vi "H3C psw cable 10G QSFP+读写操作.vi"(6 "input_psw":u8[](array[numeric]) format="%.0x", 8 "input_data":u8[](array[numeric]) format="%.0x", 9 "input_mode":string(combo), 10 "Channel":u8 max=5 step=1, 11 "VISA":refnum<visa-resource-name>="COM6") -> (0 "123equal0?":bool, 1 "result":bool, 2 "message":string, 3 "data read":u8[](array[numeric]) format="%.0x")   [LabVIEW 2011]
panel:
  out "page3 128 Bytes":u8[](array[numeric]) format="%.0x"
  out "page2 128 Bytes":u8[](array[numeric]) format="%.0x"
  out "page1 128 Bytes":u8[](array[numeric]) format="%.0x"
  in  "address":u8
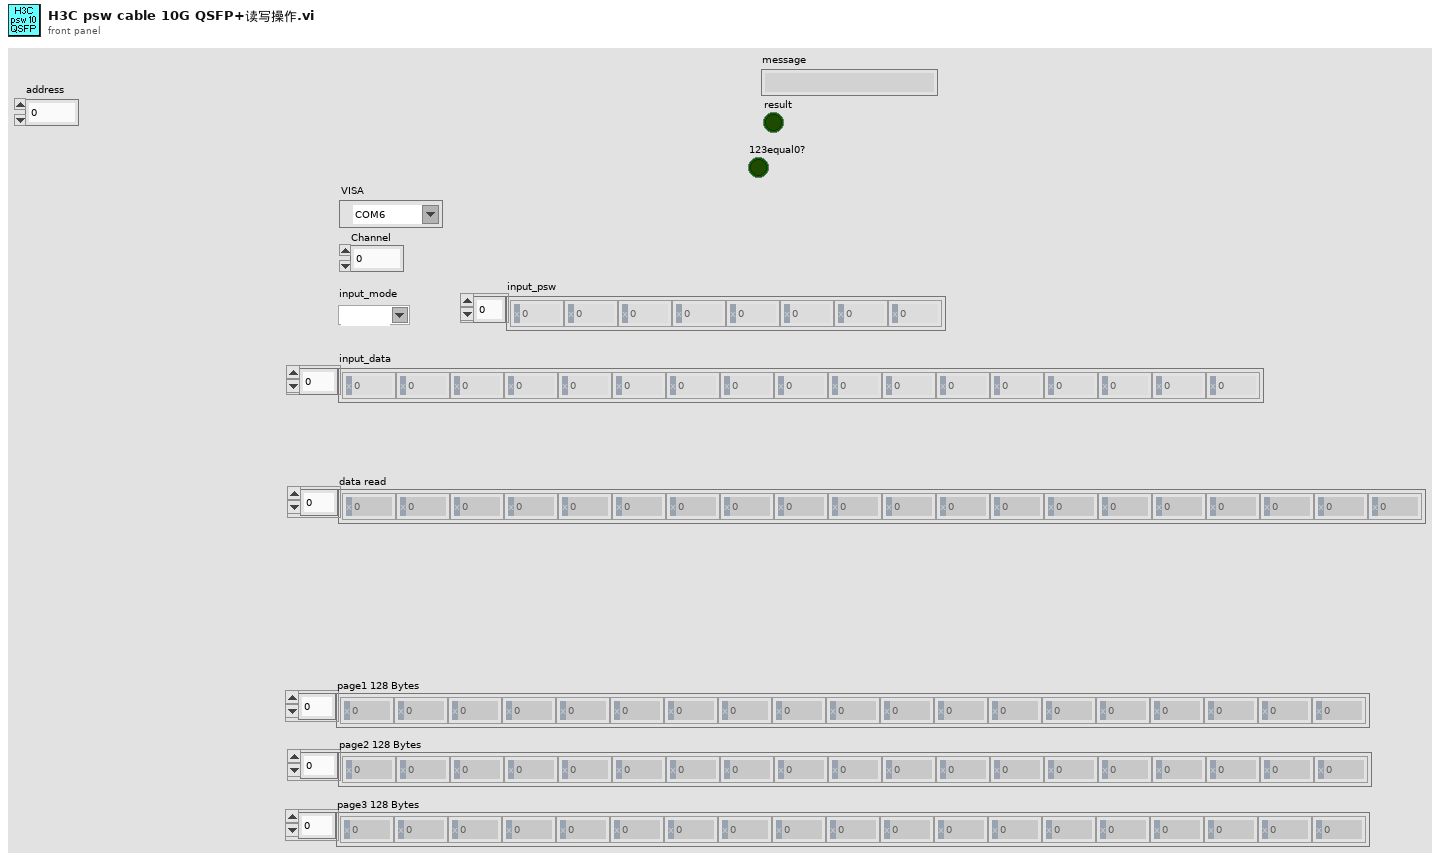
[diagram p1: front panel]
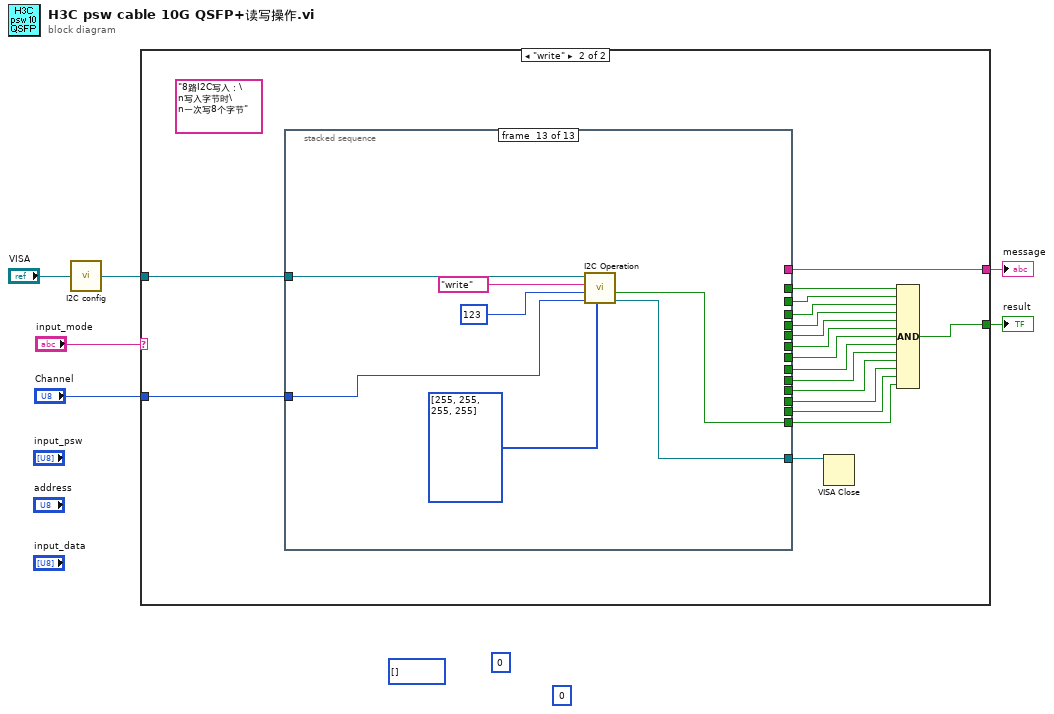
[diagram p0: block diagram]
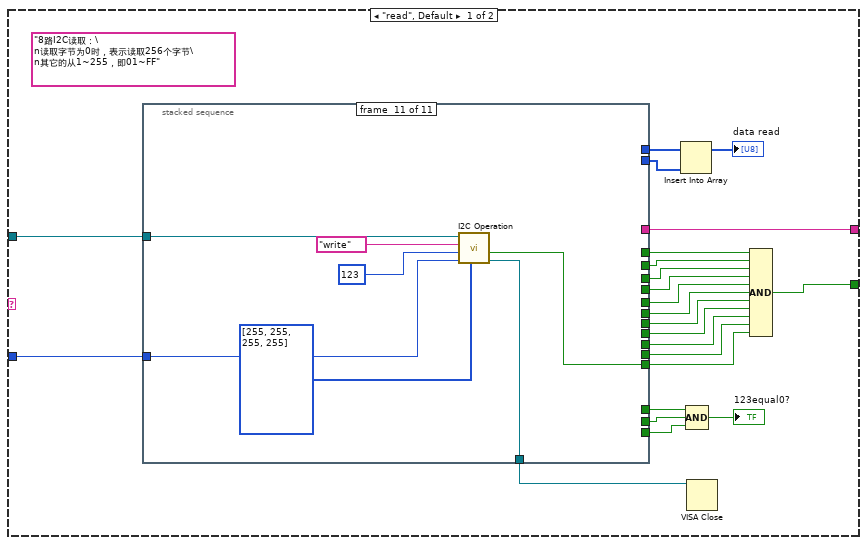
[diagram p2: hidden frame]
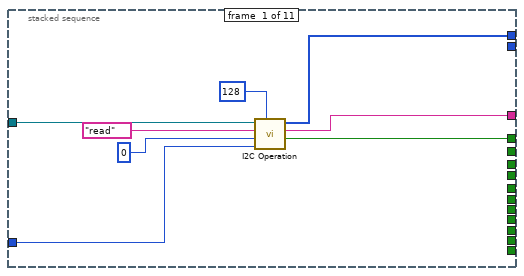
[diagram p3: hidden frame]
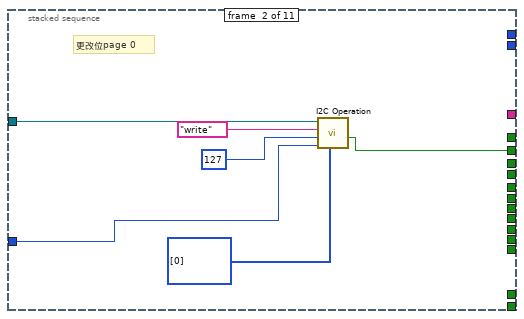
[diagram p4: hidden frame]
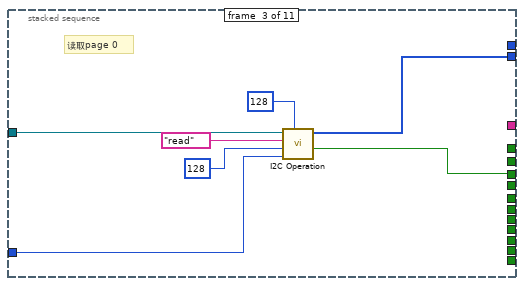
[diagram p5: hidden frame]
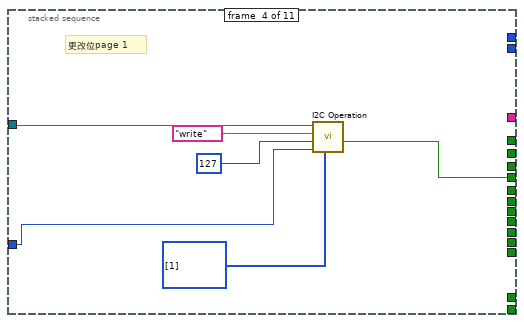
[diagram p6: hidden frame]
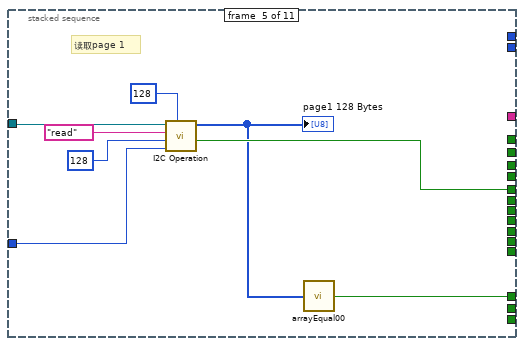
[diagram p7: hidden frame]
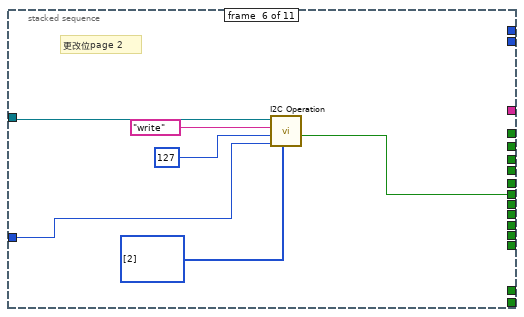
[diagram p8: hidden frame]
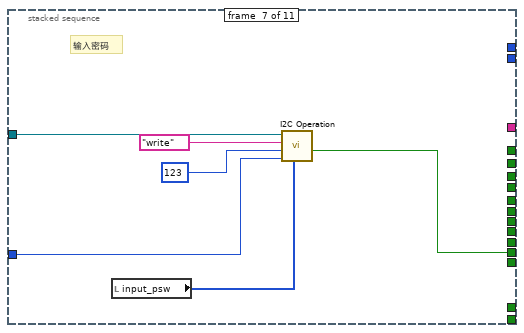
[diagram p9: hidden frame]
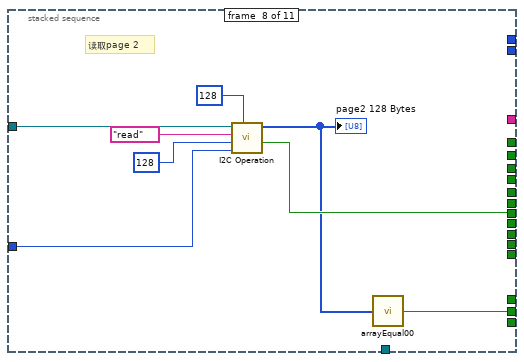
[diagram p10: hidden frame]
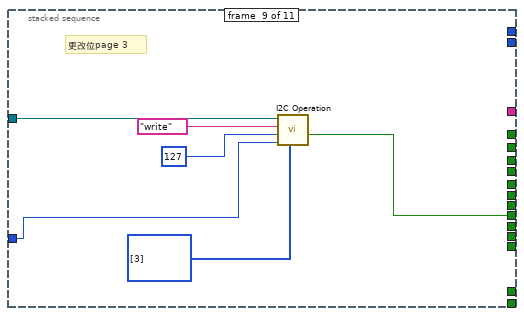
[diagram p11: hidden frame]
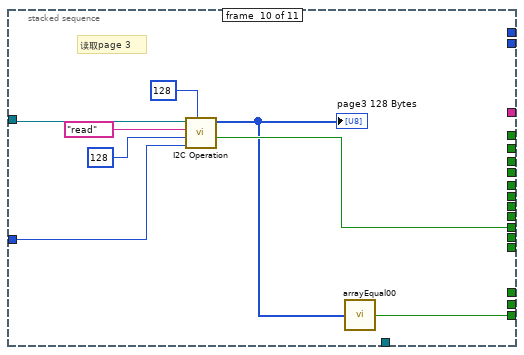
[diagram p12: hidden frame]
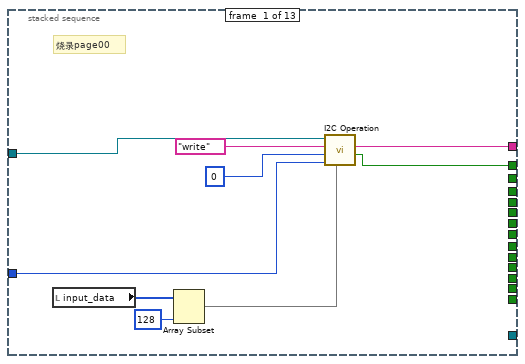
[diagram p13: hidden frame]
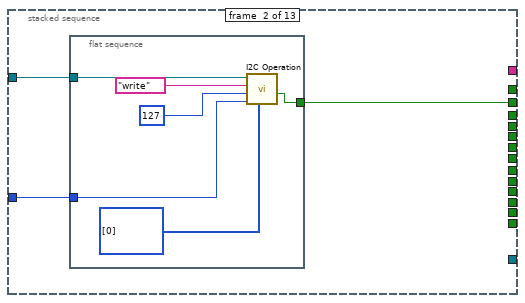
[diagram p14: hidden frame]
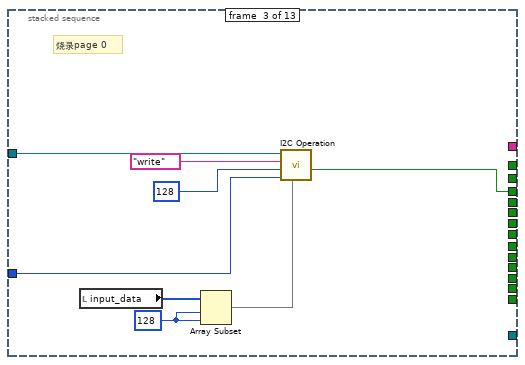
[diagram p15: hidden frame]
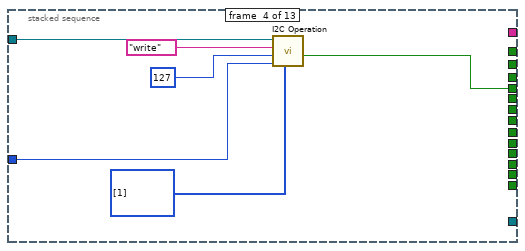
[diagram p16: hidden frame]
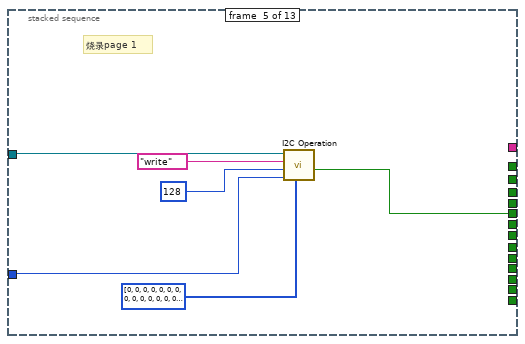
[diagram p17: hidden frame]
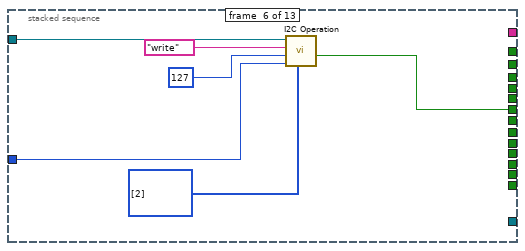
[diagram p18: hidden frame]
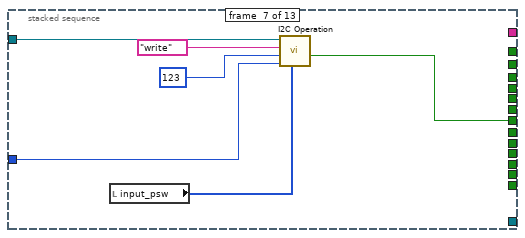
[diagram p19: hidden frame]
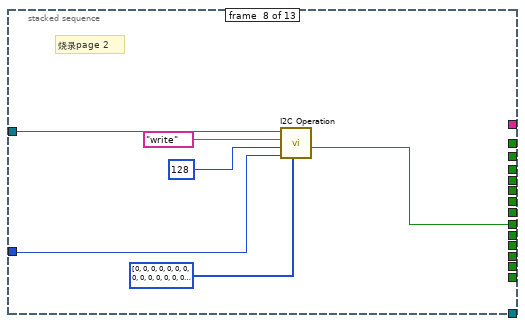
[diagram p20: hidden frame]
diagram:
  (unwired) u8[] []
  (unwired) u8 0
  (unwired) u8 0
  n1 = call "I2C config.vi"("VISA"="VISA") -> ("VISA资源名称输出"=w1:refnum<visa-resource-name>)
  n2 = case shown="\"write\"" "input_mode" {
    tunnel: w1 -> [w29 w123]
    tunnel: "Channel" -> [w28 w122]
    tunnel: [w27 w121] -> w4
    tunnel: [w14 w107] -> w3
    frame "read", Default {
      (unwired) "8路I2C读取：\n读取字节为0时，表示读取256个字节\n其它的从1~255，即01~FF"
      n3 = stacked-sequence {
        tunnel: w29 -> [w37 w40 w50 w53 w61 w67 w73 w81 w87 w95 w103]
        tunnel: w28 -> [w33 w39 w46 w52 w60 w66 w72 w80 w86 w94 w102]
        tunnel: [w32 _ _ _ _ _ _ _ _ _ _] -> w27
        tunnel: [w31 _ _ _ _ _ _ _ _ _ _] -> w23
        tunnel: [w30 _ _ _ _ _ _ _ _ _ _] -> w26
        tunnel: [_ _ w45 _ _ _ _ _ _ _ _] -> w25
        tunnel: [_ w38 _ _ _ _ _ _ _ _ _] -> w22
        tunnel: [_ _ w44 _ _ _ _ _ _ _ _] -> w21
        tunnel: [_ _ _ w51 _ _ _ _ _ _ _] -> w20
        tunnel: [_ _ _ _ w59 _ _ _ _ _ _] -> w19
        tunnel: [_ _ _ _ _ w65 _ _ _ _ _] -> w18
        tunnel: [_ _ _ _ _ _ _ w79 _ _ _] -> w17
        tunnel: [_ _ _ _ _ _ _ _ w85 _ _] -> w16
        tunnel: [_ _ _ _ _ _ _ _ _ w93 _] -> w15
        tunnel: [_ _ _ _ _ _ w71 _ _ _ _] -> w13
        tunnel: [_ _ _ _ _ _ _ _ _ _ w100] -> w12
        tunnel: [_ _ _ _ w57 _ _ _ _ _ _] -> w11
        tunnel: [_ _ _ _ _ _ _ w78 _ _ _] -> w10
        tunnel: [_ _ _ _ _ _ _ _ _ w92 _] -> w9
        tunnel: [_ _ _ _ _ _ _ _ _ _ w99] -> w7
        frame #0 {
          n4 = call "I2C Operation.vi"("size"=128, "Channel"=w33, "address"=u8 0, "mode"="read", "VISA"=w37) -> ("result"=w31:bool, "message"=w32:string, "Data Out"=w30:u8[])  [unwired: 3 in, 1 out]
        }
        frame #1 {
          # "更改位page 0"
          n5 = call "I2C Operation.vi"("input_data"=u8[] [0], "Channel"=w39, "address"=u8 127, "mode"="write", "VISA"=w40) -> ("result"=w38:bool)  [unwired: 3 in, 3 out]
        }
        frame #2 {
          # "读取page 0"
          n6 = call "I2C Operation.vi"("size"=128, "Channel"=w46, "address"=u8 128, "mode"="read", "VISA"=w50) -> ("result"=w44:bool, "Data Out"=w45:u8[])  [unwired: 3 in, 2 out]
        }
        frame #3 {
          # "更改位page 1"
          n7 = call "I2C Operation.vi"("input_data"=u8[] [1], "Channel"=w52, "address"=u8 127, "mode"="write", "VISA"=w53) -> ("result"=w51:bool)  [unwired: 3 in, 3 out]
        }
        frame #4 {
          # "读取page 1"
          n8 = call "I2C Operation.vi"("size"=128, "Channel"=w60, "address"=u8 128, "mode"="read", "VISA"=w61) -> ("result"=w59:bool, "Data Out"=w58:u8[])  [unwired: 3 in, 2 out]
          "page1 128 Bytes" <- w58
          n9 = call "arrayEqual00.vi"("input"=w58) -> ("equal"=w57:bool)
        }
        frame #5 {
          # "更改位page 2"
          n10 = call "I2C Operation.vi"("input_data"=u8[] [2], "Channel"=w66, "address"=u8 127, "mode"="write", "VISA"=w67) -> ("result"=w65:bool)  [unwired: 3 in, 3 out]
        }
        frame #6 {
          # "输入密码"
          n11 = local read "input_psw"() -> (w74:u8[])
          n12 = call "I2C Operation.vi"("input_data"=w74, "Channel"=w72, "address"=u8 123, "mode"="write", "VISA"=w73) -> ("result"=w71:bool)  [unwired: 3 in, 3 out]
        }
        frame #7 {
          # "读取page 2"
          n13 = call "I2C Operation.vi"("size"=128, "Channel"=w80, "address"=u8 128, "mode"="read", "VISA"=w81) -> ("result"=w79:bool, "Data Out"=w77:u8[])  [unwired: 3 in, 2 out]
          "page2 128 Bytes" <- w77
          n14 = call "arrayEqual00.vi"("input"=w77) -> ("equal"=w78:bool)
        }
        frame #8 {
          # "更改位page 3"
          n15 = call "I2C Operation.vi"("input_data"=u8[] [3], "Channel"=w86, "address"=u8 127, "mode"="write", "VISA"=w87) -> ("result"=w85:bool)  [unwired: 3 in, 3 out]
        }
        frame #9 {
          # "读取page 3"
          n16 = call "I2C Operation.vi"("size"=128, "Channel"=w94, "address"=u8 128, "mode"="read", "VISA"=w95) -> ("result"=w93:bool, "Data Out"=w91:u8[])  [unwired: 3 in, 2 out]
          "page3 128 Bytes" <- w91
          n17 = call "arrayEqual00.vi"("input"=w91) -> ("equal"=w92:bool)
        }
        frame #10 {
          n18 = call "I2C Operation.vi"("input_data"=u8[] [255, 255, 255, 255], "Channel"=w102, "address"=u8 123, "mode"="write", "VISA"=w103) -> ("VISA  2"=w99:refnum<visa-resource-name>, "result"=w100:bool)  [unwired: 3 in, 2 out]
        }
      }
      n19 = Insert Into Array(array=w26, new element=w25) -> (→"data read":u8[])  [unwired: 1 in]
      n20 = Compound Arithmetic op=AND(w11, w10, w9) -> (→"123equal0?":bool)
      n21 = VISA Close(VISA resource name=w7) -> ()  [unwired: 1 in, 1 out]
      n22 = Compound Arithmetic op=AND(w23, w22, w21, w20, w19, w18, w17, w16, w15, w13, w12) -> (w14:bool)
    }
    frame "write" {
      (unwired) "8路I2C写入：\n写入字节时\n一次写8个字节"
      n23 = stacked-sequence {
        tunnel: w123 -> [w132 w135 w149 w151 w158 w164 w170 w176 w181 w188 w195 w201 w208]
        tunnel: w122 -> [w130 w134 w147 w152 w157 w165 w171 w175 w182 w187 w194 w200 w207]
        tunnel: [w129 _ _ _ _ _ _ _ _ _ _ _ _] -> w121
        tunnel: [w128 _ _ _ _ _ _ _ _ _ _ _ _] -> w120
        tunnel: [_ w133 _ _ _ _ _ _ _ _ _ _ _] -> w119
        tunnel: [_ _ w145 _ _ _ _ _ _ _ _ _ _] -> w118
        tunnel: [_ _ _ w150 _ _ _ _ _ _ _ _ _] -> w117
        tunnel: [_ _ _ _ w156 _ _ _ _ _ _ _ _] -> w116
        tunnel: [_ _ _ _ _ w162 _ _ _ _ _ _ _] -> w115
        tunnel: [_ _ _ _ _ _ w168 _ _ _ _ _ _] -> w114
        tunnel: [_ _ _ _ _ _ _ w174 _ _ _ _ _] -> w113
        tunnel: [_ _ _ _ _ _ _ _ w180 _ _ _ _] -> w112
        tunnel: [_ _ _ _ _ _ _ _ _ w186 _ _ _] -> w111
        tunnel: [_ _ _ _ _ _ _ _ _ _ w192 _ _] -> w110
        tunnel: [_ _ _ _ _ _ _ _ _ _ _ w198 _] -> w109
        tunnel: [_ _ _ _ _ _ _ _ _ _ _ _ w205] -> w108
        tunnel: [_ _ _ _ _ _ _ _ _ _ _ _ w204] -> w106
        frame #0 {
          # "烧录page00"
          n24 = local read "input_data"() -> (w126:u8[])
          n25 = Array Subset(array=w126, length=128 ("长度")) -> (w124:u8[])  [unwired: 1 in]
          n26 = call "I2C Operation.vi"("input_data"=w124, "Channel"=w130, "address"=u8 0, "mode"="write", "VISA"=w132) -> ("result"=w128:bool, "message"=w129:string)  [unwired: 3 in, 2 out]
        }
        frame #1 {
          n27 = flat-sequence {
            tunnel: [w136] -> w133
            tunnel: w135 -> [w141]
            tunnel: w134 -> [w139]
            frame #0 {
              n28 = call "I2C Operation.vi"("input_data"=u8[] [0], "Channel"=w139, "address"=u8 127, "mode"="write", "VISA"=w141) -> ("result"=w136:bool)  [unwired: 3 in, 3 out]
            }
          }
        }
        frame #2 {
          w144 = 128 ("长度")
          # "烧录page 0"
          n29 = local read "input_data"() -> (w143:u8[])
          n30 = Array Subset(array=w143, index=w144, length=w144) -> (w142:u8[])
          n31 = call "I2C Operation.vi"("input_data"=w142, "Channel"=w147, "address"=u8 128, "mode"="write", "VISA"=w149) -> ("result"=w145:bool)  [unwired: 3 in, 3 out]
        }
        frame #3 {
          n32 = call "I2C Operation.vi"("input_data"=u8[] [1], "Channel"=w152, "address"=u8 127, "mode"="write", "VISA"=w151) -> ("result"=w150:bool)  [unwired: 3 in, 3 out]
        }
        frame #4 {
          # "烧录page 1"
          n33 = call "I2C Operation.vi"("input_data"=u8[] [0, 0, 0, 0, 0, 0, 0, 0, 0, 0, 0, 0, 0, 0, 0, 0, 0, 0, 0, 0, 0, 0, 0, 0, 0, 0, 0, 0, 0, 0, 0, 0, 0, 0, 0, 0, 0, 0, 0, 0, 0, 0, 0, 0, 0, 0, 0, 0, 0, 0, 0, 0, 0, 0, 0, 0, 0, 0, 0, 0, 0, 0, 0, 0, 0, 0, 0, 0, 0, 0, 0, 0, 0, 0, 0, 0, 0, 0, 0, 0, 0, 0, 0, 0, 0, 0, 0, 0, 0, 0, 0, 0, 0, 0, 0, 0, 0, 0, 0, 0, 0, 0, 0, 0, 0, 0, 0, 0, 0, 0, 0, 0, 0, 0, 0, 0, 0, 0, 0, 0, 0, 0, 0, 0, 0, 0, 0, 0], "Channel"=w157, "address"=u8 128, "mode"="write", "VISA"=w158) -> ("result"=w156:bool)  [unwired: 3 in, 3 out]
        }
        frame #5 {
          n34 = call "I2C Operation.vi"("input_data"=u8[] [2], "Channel"=w165, "address"=u8 127, "mode"="write", "VISA"=w164) -> ("result"=w162:bool)  [unwired: 3 in, 3 out]
        }
        frame #6 {
          n35 = local read "input_psw"() -> (w169:u8[])
          n36 = call "I2C Operation.vi"("input_data"=w169, "Channel"=w171, "address"=u8 123, "mode"="write", "VISA"=w170) -> ("result"=w168:bool)  [unwired: 3 in, 3 out]
        }
        frame #7 {
          # "烧录page 2"
          n37 = call "I2C Operation.vi"("input_data"=u8[] [0, 0, 0, 0, 0, 0, 0, 0, 0, 0, 0, 0, 0, 0, 0, 0, 0, 0, 0, 0, 0, 0, 0, 0, 0, 0, 0, 0, 0, 0, 0, 0, 0, 0, 0, 0, 0, 0, 0, 0, 0, 0, 0, 0, 0, 0, 0, 0, 0, 0, 0, 0, 0, 0, 0, 0, 0, 0, 0, 0, 0, 0, 0, 0, 0, 0, 0, 0, 0, 0, 0, 0, 0, 0, 0, 0, 0, 0, 0, 0, 0, 0, 0, 0, 0, 0, 0, 0, 0, 0, 0, 0, 0, 0, 0, 0, 0, 0, 0, 0, 0, 0, 0, 0, 0, 0, 0, 0, 0, 0, 0, 0, 0, 0, 0, 0, 0, 0, 0, 0, 0, 0, 0, 0, 0, 0, 0, 0], "Channel"=w175, "address"=u8 128, "mode"="write", "VISA"=w176) -> ("result"=w174:bool)  [unwired: 3 in, 3 out]
        }
        frame #8 {
          n38 = call "I2C Operation.vi"("input_data"=u8[] [3], "Channel"=w182, "address"=u8 127, "mode"="write", "VISA"=w181) -> ("result"=w180:bool)  [unwired: 3 in, 3 out]
        }
        frame #9 {
          # "烧录page 3"
          n39 = call "I2C Operation.vi"("input_data"=u8[] [0, 0, 0, 0, 0, 0, 0, 0, 0, 0, 0, 0, 0, 0, 0, 0, 0, 0, 0, 0, 0, 0, 0, 0, 0, 0, 0, 0, 0, 0, 0, 0, 0, 0, 0, 0, 0, 0, 0, 0, 0, 0, 0, 0, 0, 0, 0, 0, 0, 0, 0, 0, 0, 0, 0, 0, 0, 0, 0, 0, 0, 0, 0, 0, 0, 0, 0, 0, 0, 0, 0, 0, 0, 0, 0, 0, 0, 0, 0, 0, 0, 0, 0, 0, 0, 0, 0, 0, 0, 0, 0, 0, 0, 0, 0, 0, 0, 0, 0, 0, 0, 0, 0, 0, 0, 0, 0, 0, 0, 0, 0, 0, 0, 0, 0, 0, 0, 0, 0, 0, 0, 0, 0, 0, 0, 0, 0, 0], "Channel"=w187, "address"=u8 128, "mode"="write", "VISA"=w188) -> ("result"=w186:bool)  [unwired: 3 in, 3 out]
        }
        frame #10 {
          n40 = call "I2C Operation.vi"("input_data"=u8[] [0], "Channel"=w194, "address"=u8 127, "mode"="write", "VISA"=w195) -> ("result"=w192:bool)  [unwired: 3 in, 3 out]
        }
        frame #11 {
          n41 = call "I2C Operation.vi"("input_data"=u8[] [226, 23, 130, 37], "Channel"=w200, "address"=u8 123, "mode"="write", "VISA"=w201) -> ("result"=w198:bool)  [unwired: 3 in, 3 out]
        }
        frame #12 {
          n42 = call "I2C Operation.vi"("input_data"=u8[] [255, 255, 255, 255], "Channel"=w207, "address"=u8 123, "mode"="write", "VISA"=w208) -> ("VISA  2"=w204:refnum<visa-resource-name>, "result"=w205:bool)  [unwired: 3 in, 2 out]
        }
      }
      n43 = VISA Close(VISA resource name=w106) -> ()  [unwired: 1 in, 1 out]
      n44 = Compound Arithmetic op=AND(w120, w119, w118, w117, w116, w115, w114, w113, w112, w111, w110, w109, w108) -> (w107:bool)
    }
  }
  "message" <- w4
  "result" <- w3
